vi "GenCM-Set Ring Text.vi"(0 "slot ctl refs":refnum<vi>[](array[refnum]), 7 "Output List":string[](array[string]), 9 "Input List":string[](array[string]), 11 "error in (no error)":errorcluster) -> (15 "error out":errorcluster)   [LabVIEW 2015]
uses:
  Type Defs/General PXISlot XControl/PXISlotGP.xctl
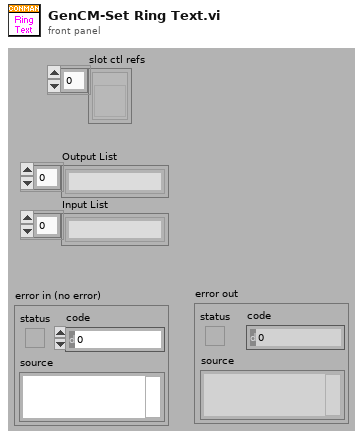
[diagram p1: front panel]
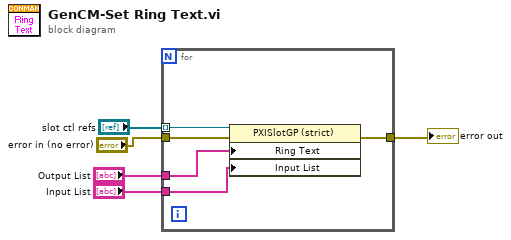
[diagram p0: block diagram]
diagram:
  n1 = for {
    tunnel: "slot ctl refs" -> [w10] mode=indexing
    tunnel: "error in (no error)" -> [w9]
    tunnel: "Output List" -> [w8]
    tunnel: [w7] -> w2
    tunnel: "Input List" -> [w6]
    n2 = property class="PXISlotGP (strict)"(reference=w10, error in=w9, "Ring Text"=w8, "Input List"=w6) -> (error out=w7:errorcluster)  [unwired: 1 out]
  }
  "error out" <- w2
